vi "Update Method Results.vi"(8 "error in (no error)":errorcluster, 10 "Method Result":refnum<class "Method Result.lvclass">, 11 "Result Table in":refnum<class "Result Table.lvclass">) -> (0 "error out":errorcluster, 1 "Result Texts":string[](array[string]), 2 "Method Result Out":refnum<class "Method Result.lvclass">, 3 "Result Table out":refnum<class "Result Table.lvclass">)   [LabVIEW 2020, in "Result Table.lvclass"]
uses:
  Result Table.lvclass
  Result Classes/Method Result/Method Result.lvclass
  Result Classes/Method Result/Method Result.lvclass/Method Result.ctl
  Result Table.lvclass/Result Table.ctl
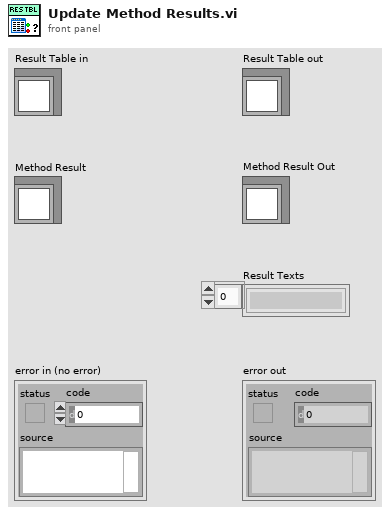
[diagram p1: front panel]
types:
  T1 = typedef "Assertion Result.lvclass/Status.ctl" = enum16{"Pass", "Fail", "Error", "Skipped", "Setup Error", "Broken", "Teardown Error"}
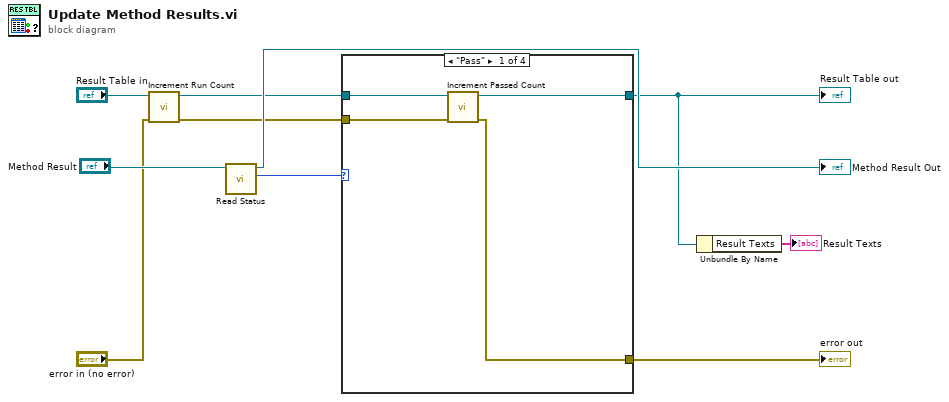
[diagram p0: block diagram]
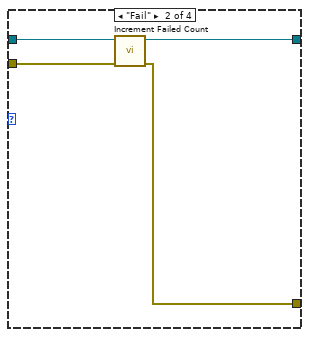
[diagram p2: hidden frame]
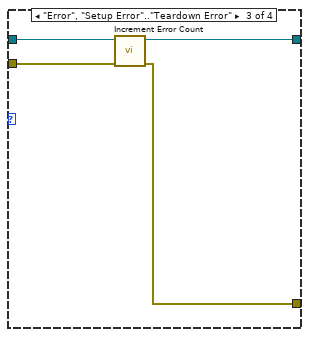
[diagram p3: hidden frame]
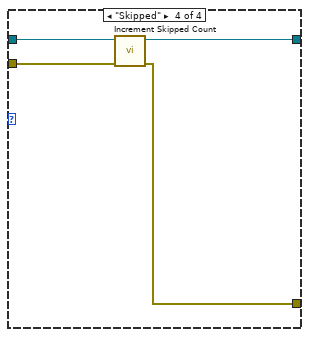
[diagram p4: hidden frame]
diagram:
  n1 = call "Increment Run Count.vi"("error in (no error)"="error in (no error)", "Result Table.lvclass"="Result Table in") -> ("error out"=w3:errorcluster, "Result Table"=w5:refnum<class "Result Table.lvclass">)  [unwired: 8 in]
  n2 = call "Read Status.vi"("Method Result In"="Method Result") -> ("Status"=w7:T1, "Method Result Out"=→"Method Result Out":refnum<class "Method Result.lvclass">)  [unwired: 8 in, 1 out]
  n3 = case shown="\"Pass\"" w7 {
    tunnel: w5 -> [w14 w18 w22 w26]
    tunnel: [w13 w17 w21 w25] -> w2
    tunnel: [w12 w16 w20 w24] -> w9
    tunnel: w3 -> [w11 w15 w19 w23]
    frame "Pass" {
      n4 = call "Increment Passed Count.vi"("error in (no error)"=w11, "Result Table.lvclass"=w14) -> ("error out"=w12:errorcluster, "Result Table"=w13:refnum<class "Result Table.lvclass">)  [unwired: 8 in]
    }
    frame "Fail" {
      n5 = call "Increment Failed Count.vi"("error in (no error)"=w15, "Result Table.lvclass"=w18) -> ("error out"=w16:errorcluster, "Result Table"=w17:refnum<class "Result Table.lvclass">)  [unwired: 8 in]
    }
    frame "Error", "Setup Error".."Teardown Error" {
      n6 = call "Increment Error Count.vi"("error in (no error)"=w19, "Result Table.lvclass"=w22) -> ("error out"=w20:errorcluster, "Result Table"=w21:refnum<class "Result Table.lvclass">)  [unwired: 8 in]
    }
    frame "Skipped" {
      n7 = call "Increment Skipped Count.vi"("error in (no error)"=w23, "Result Table.lvclass"=w26) -> ("error out"=w24:errorcluster, "Result Table"=w25:refnum<class "Result Table.lvclass">)  [unwired: 8 in]
    }
  }
  "error out" <- w9
  "Result Table out" <- w2
  n8 = Unbundle By Name(w2) -> ("Result Texts"=→"Result Texts":string[])
